vi "3.vi"(7 "Kezelõpult":T1={"Filt_alsó"=750.0, "Filt_felsõ"=7400.0, "Optikai elem hossza (km)"=0.000445, "Referencia hullámhossz (nm)"=800.0, " Illesztendõ polinom fokszáma"=7, "Megjegyzések"=""}, 8 "error in (no error)":errorcluster, 11 "adat":T2) -> (0 "error out":errorcluster, 1 "XY Graph 5":cluster{dbl[], dbl[]}[](graph), 2 "XY Graph 4":cluster{dbl[], dbl[]}[](graph), 3 "XY Graph 3":cluster{dbl[], dbl[]}[](graph), 5 "Fázisderiváltak":dbl[](array[numeric]))   [LabVIEW 2023]
doc: "Folytonos spektrális fázisfüggvény elõállítása, polinom illesztése, fázisderiváltak és diszperziós görbe meghatározása."
uses:
  adat.ctl
  control panel.ctl
  <vilib>/Analysis/NI_AALPro.lvlib
  <vilib>/gmath/NI_Gmath.lvlib
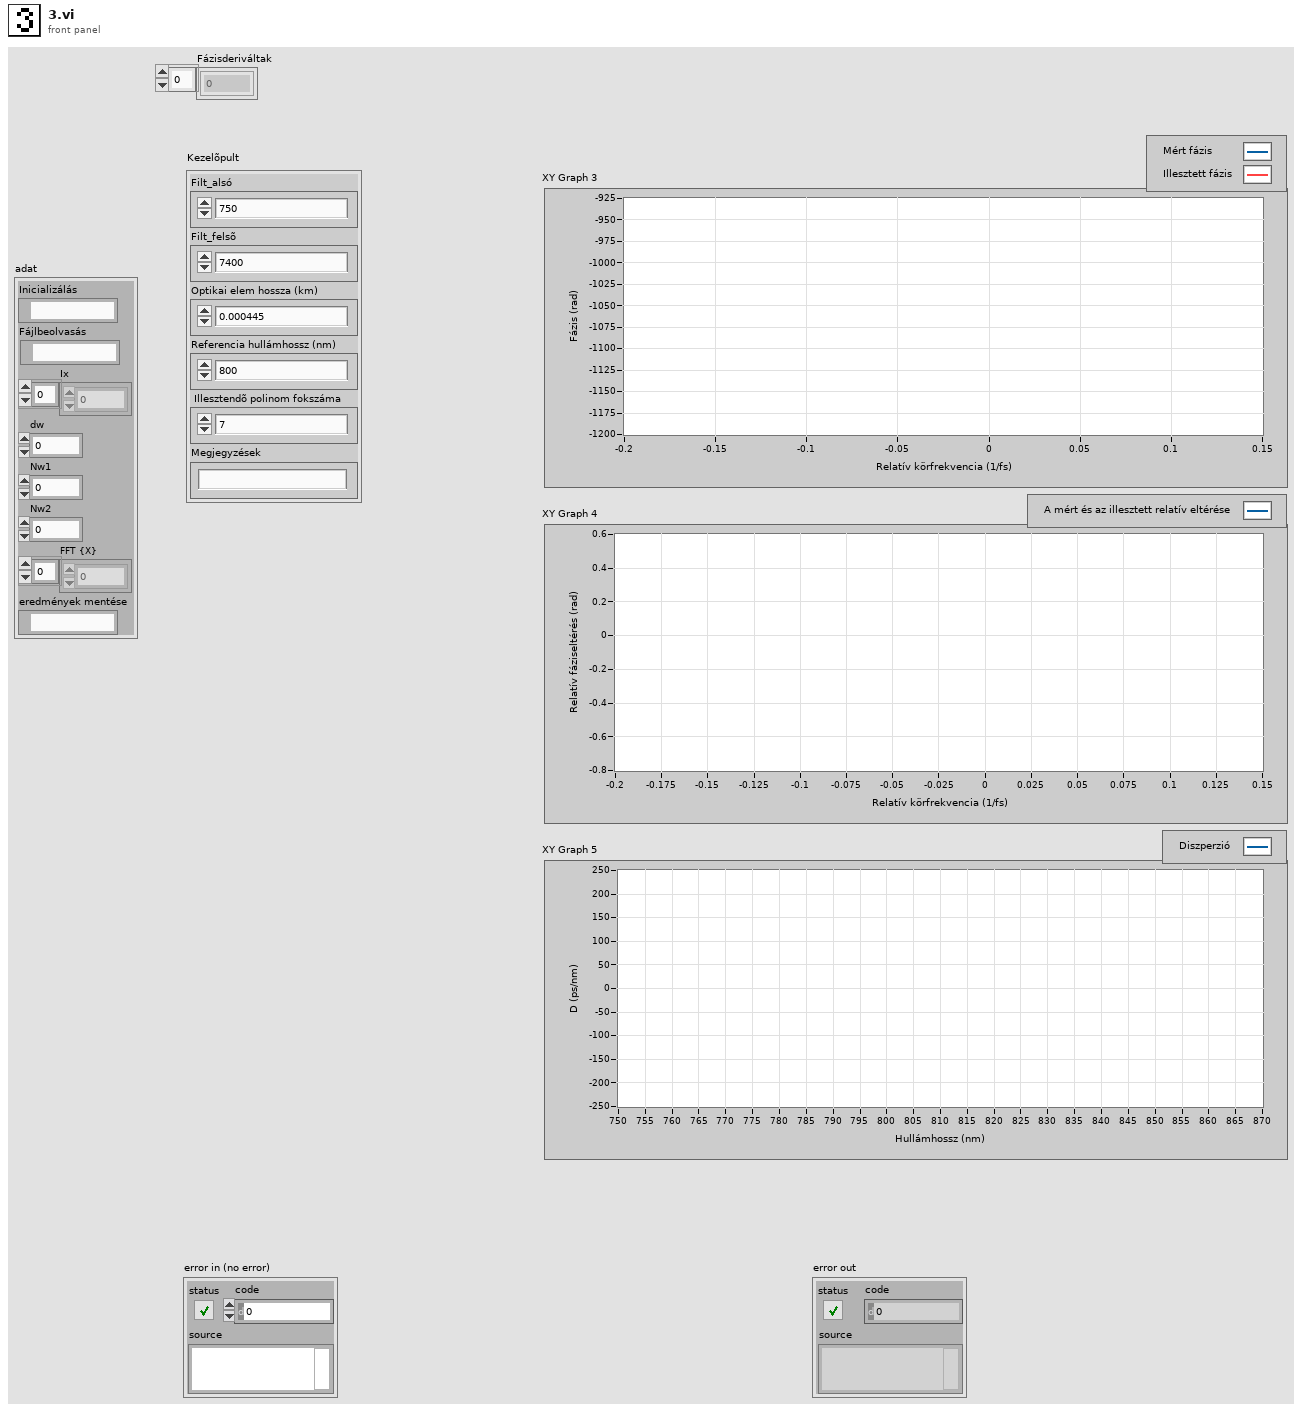
[diagram p1: front panel]
types:
  T1 = typedef "control panel.ctl" = cluster{"Filt_alsó":dbl, "Filt_felsõ":dbl, "Optikai elem hossza (km)":dbl, "Referencia hullámhossz (nm)":dbl, " Illesztendõ polinom fokszáma":i32, "Megjegyzések":string}
  T2 = typedef "adat.ctl" = cluster{"Inicializálás":path, "Fájlbeolvasás":path, "Ix":dbl[], "dw":dbl, "Nw1":dbl, "Nw2":dbl, "FFT {X}":cdb[], "eredmények mentése":path}
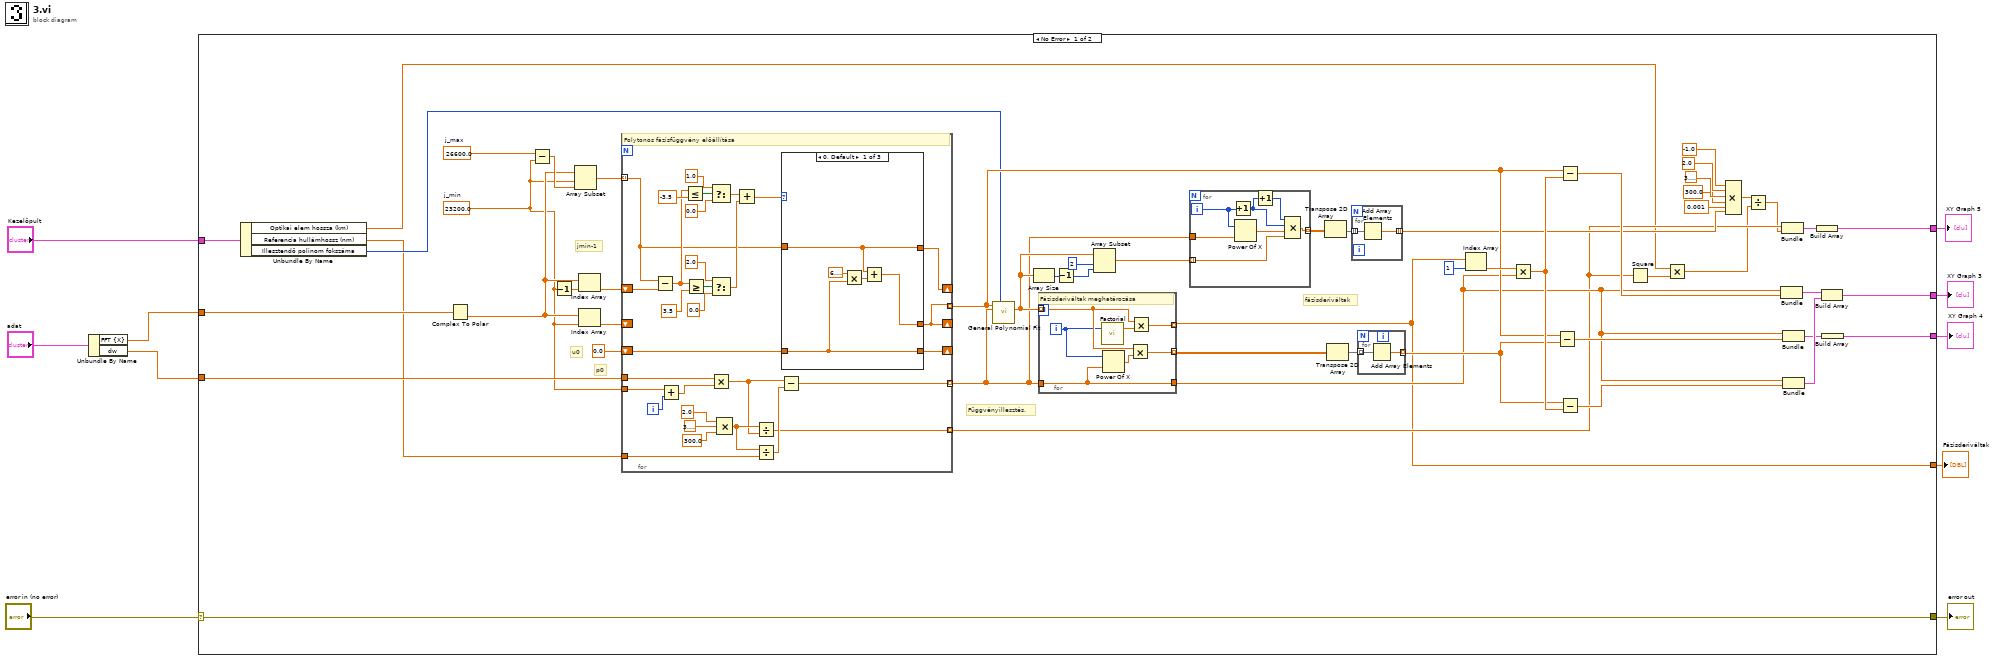
[diagram p0: block diagram]
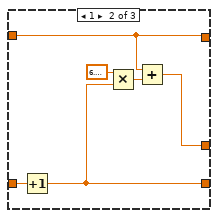
[diagram p2: hidden frame]
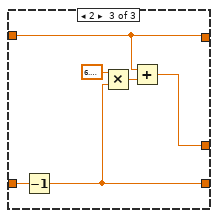
[diagram p3: hidden frame]
diagram:
  n1 = Unbundle By Name("adat") -> ("FFT {X}"=w3:cdb[], "dw"=w4:dbl)
  n2 = case shown="No Error" "error in (no error)" {
    selector: "error in (no error)" -> [w16 w131]
    tunnel: [w62 _] -> w10
    tunnel: [w11 _] -> w9
    tunnel: w4 -> [w57 _]
    tunnel: w3 -> [w55 _]
    tunnel: [w13 _] -> w8
    tunnel: "Kezelõpult" -> [w20 _]
    tunnel: [w16 w131] -> w6
    tunnel: [w15 _] -> w2
    frame No Error {
      w22 = 26600.0  # j_max
      w21 = 23200.0  # j_min
      # "fázisderiváltak"
      # "Függvényillesztés."
      # "jmin-1"
      # "u0"
      # "p0"
      n3 = Unbundle By Name(w20) -> ("Optikai elem hossza (km)"=w17:dbl, "Referencia hullámhossz (nm)"=w18:dbl, "Illesztendõ polinom fokszáma"=w19:i32)
      n4 = Complex To Polar(r * e^(i*theta)=w55) -> (theta=w52:dbl[])  [unwired: 1 out]
      n5 = Subtract(x=w22, y=w21) -> (x-y=w54:dbl)
      n6 = Decrement(x=w21) -> (x-1=w51:dbl)
      n7 = Array Subset(array=w52, index=w21, length=w54) -> (w53:dbl[])
      n8 = Index Array(array=w52, index=w51) -> (element=w49:dbl)
      n9 = Index Array(array=w52, index=w21) -> (element=w50:dbl)
      n10 = for {
        shift-right: [w93] -> _
        shift-left: w50 -> [_]
        shift-right: [w94] -> _
        shift-left: 0.0 -> [w95]
        tunnel: w53 -> [w91] mode=indexing
        tunnel: [w93] -> w48 mode=indexing
        shift-right: [w92] -> _
        shift-left: w49 -> [w90]
        tunnel: w57 -> [w86]
        tunnel: w21 -> [w84]
        tunnel: [w83] -> w38 mode=indexing
        tunnel: [w79] -> w26 mode=indexing
        tunnel: w18 -> [w78]
        i -> [w85]
        # "Folytonos fázisfüggvény elõállítása"
        n11 = Subtract(x=w91, y=w90) -> (x-y=w104:dbl)
        n12 = Add(x=w84, y=w85) -> (x+y=w77:dbl)
        n13 = Less Or Equal?(x=w104, y=-3.5) -> (x <= y?=w103:bool)
        n14 = Greater Or Equal?(x=w104, y=3.5) -> (x >= y?=w100:bool)
        n15 = Select(t=1.0, s=w103, f=0.0 ("t")) -> (s? t:f=w97:dbl)
        n16 = Select(t=2.0, s=w100, f=0.0 ("t")) -> (s? t:f=w96:dbl)
        n17 = Multiply(x=w86, y=w77) -> (x*y=w80:dbl)
        n18 = Compound Arithmetic op=MULTIPLY(2.0 ("value"), 3.141592653589793, 300.0 ("value")) -> (w81:dbl)
        n19 = Add(x=w97, y=w96) -> (x+y=w76:dbl)
        n20 = Divide(x=w81, y=w80) -> (x/y=w79:dbl)
        n21 = Divide(x=w81, y=w78) -> (x/y=w82:dbl)
        n22 = Subtract(x=w80, y=w82) -> (x-y=w83:dbl)
        n23 = case shown="0, Default" w76 {
          tunnel: w91 -> [w107 w112 w118]
          tunnel: w95 -> [w108 w117 w123]
          tunnel: [w108 w114 w119] -> w94
          tunnel: [w109 w113 w120] -> w93
          tunnel: [w107 w112 w118] -> w92
          frame 0, Default {
            n24 = Multiply(x=6.283185307179586, y=w108) -> (x*y=w111:dbl)
            n25 = Add(x=w107, y=w111) -> (x+y=w109:dbl)
          }
          frame 1 {
            n26 = Increment(x=w117) -> (x+1=w114:dbl)
            n27 = Multiply(x=6.283185307179586, y=w114) -> (x*y=w116:dbl)
            n28 = Add(x=w112, y=w116) -> (x+y=w113:dbl)
          }
          frame 2 {
            n29 = Decrement(x=w123) -> (x-1=w119:dbl)
            n30 = Multiply(x=6.283185307179586, y=w119) -> (x*y=w122:dbl)
            n31 = Add(x=w118, y=w122) -> (x+y=w120:dbl)
          }
        }
      }
      n32 = call <vilib>:"General Polynomial Fit.vi"("Y"=w48, "polynomial order"=w19, "X"=w38) -> ("Polynomial Coefficients"=w43:dbl[])  [unwired: 9 in, 3 out]
      n33 = Array Size(array=w43) -> (size(s)=w42:i32)
      n34 = for {
        tunnel: w43 -> [w127] mode=indexing
        tunnel: [w129] -> w15 mode=indexing
        tunnel: w38 -> [w126]
        tunnel: [w126] -> w34
        tunnel: [w125] -> w46 mode=indexing
        i -> [w124]
        # "Fázisderiváltak meghatározása"
        n35 = call <vilib>:"Factorial.vi"("n"=w124) -> ("n!"=w130:dbl)  [unwired: 2 in]
        n36 = Power Of X(1:w126, 2:w124) -> (0:w128:dbl[])
        n37 = Multiply(x=w127, y=w128) -> (x*y=w125:dbl[])
        n38 = Multiply(x=w127, y=w130) -> (x*y=w129:dbl)
      }
      n39 = Decrement(x=w42) -> (x-1=w41:i32)
      n40 = Array Subset(array=w43, index=2, length=w41) -> (w39:dbl[])
      n41 = for {
        tunnel: w39 -> [w71] mode=indexing
        tunnel: w38 -> [w73]
        tunnel: [w70] -> w37 mode=indexing
        i -> [w67]
        n42 = Increment(x=w67) -> (x+1=w68:i32)
        n43 = Power Of X(1:w73, 2:w67) -> (0:w72:dbl[])
        n44 = Increment(x=w68) -> (x+1=w69:i32)
        n45 = Compound Arithmetic op=MULTIPLY(w69, w68, w72, w71) -> (w70:dbl[])
      }
      n46 = Transpose 2D Array(2D array=w37) -> (transposed array=w36:dbl[][])
      n47 = Transpose 2D Array(2D array=w46) -> (transposed array=w45:dbl[][])
      n48 = for {
        tunnel: w36 -> [w66] mode=indexing
        tunnel: [w65] -> w28 mode=indexing
        n49 = Add Array Elements(numeric array=w66) -> (sum=w65:dbl)
      }
      n50 = for {
        tunnel: w45 -> [w75] mode=indexing
        tunnel: [w74] -> w44 mode=indexing
        n51 = Add Array Elements(numeric array=w75) -> (sum=w74:dbl)
      }
      n52 = Index Array(array=w15, index=1) -> (element=w64:dbl)
      n53 = Multiply(x=w64, y=w34) -> (x*y=w63:dbl[])
      n54 = Subtract(x=w48, y=w44) -> (x-y=w47:dbl[])
      n55 = Subtract(x=w48, y=w63) -> (x-y=w59:dbl[])
      n56 = Subtract(x=w44, y=w63) -> (x-y=w61:dbl[])
      n57 = Square(x=w26) -> (x^2=w25:dbl[])
      n58 = Multiply(x=w17, y=w25) -> (x*y=w24:dbl[])
      n59 = Compound Arithmetic op=MULTIPLY(-1.0 ("value"), 2.0 ("value"), 3.141592653589793, 300.0 ("value"), 0.001 ("value"), w28) -> (w27:dbl[])
      n60 = Divide(x=w27, y=w24) -> (x/y=w23:dbl[])
      n61 = Bundle(w34, w59) -> (w60:cluster{dbl[], dbl[]})  [unwired: 1 in]
      n62 = Bundle(w26, w23) -> (w14:cluster{dbl[], dbl[]})  [unwired: 1 in]
      n63 = Bundle(w34, w47) -> (w12:cluster{dbl[], dbl[]})  [unwired: 1 in]
      n64 = Bundle(w34, w61) -> (w58:cluster{dbl[], dbl[]})  [unwired: 1 in]
      n65 = Build Array(w14) -> (w13:cluster{dbl[], dbl[]}[])
      n66 = Build Array(w60, w58) -> (w62:cluster{dbl[], dbl[]}[])
      n67 = Build Array(w12) -> (w11:cluster{dbl[], dbl[]}[])
    }
    frame Error {
    }
  }
  "XY Graph 3" <- w10
  "XY Graph 4" <- w9
  "XY Graph 5" <- w8
  "error out" <- w6
  "Fázisderiváltak" <- w2
